vi "Kinematics.vi"() -> ()   [LabVIEW 2024]
panel:
  in  "Lengths":cluster{"L 1":dbl, "L 2":dbl}={"L 1"=80.0, "L 2"=115.0} {"L 2" scale=0.0..200.0; "L 1" scale=0.0..200.0}
  in  "2D Pict origin":cluster{"x":dbl, "y":dbl}={"x"=80.0, "y"=350.0}
  out "2D Picture":picture
  in  "Positions":cluster{dbl, dbl}[](array[cluster]) {"?" format="%.1f"; "?" format="%#.1f"}
  # "mm"
  # "mm"
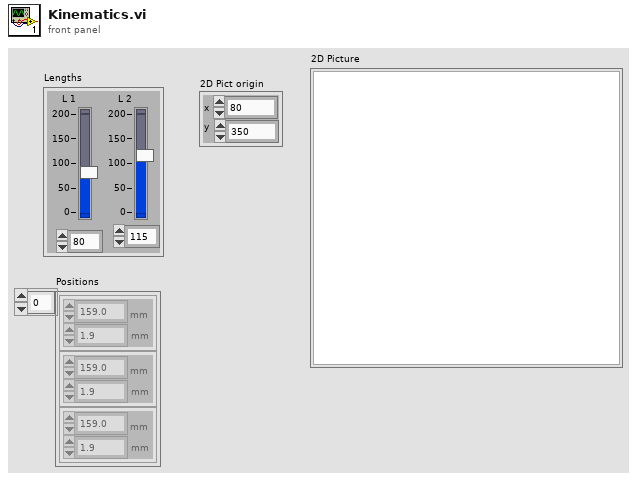
[diagram p1: front panel]
types:
  T1 = cluster{"Width":u16, "Style":enum32{"Solid", "Dash", "Dot", "DashDot", "DashDotDot"}}
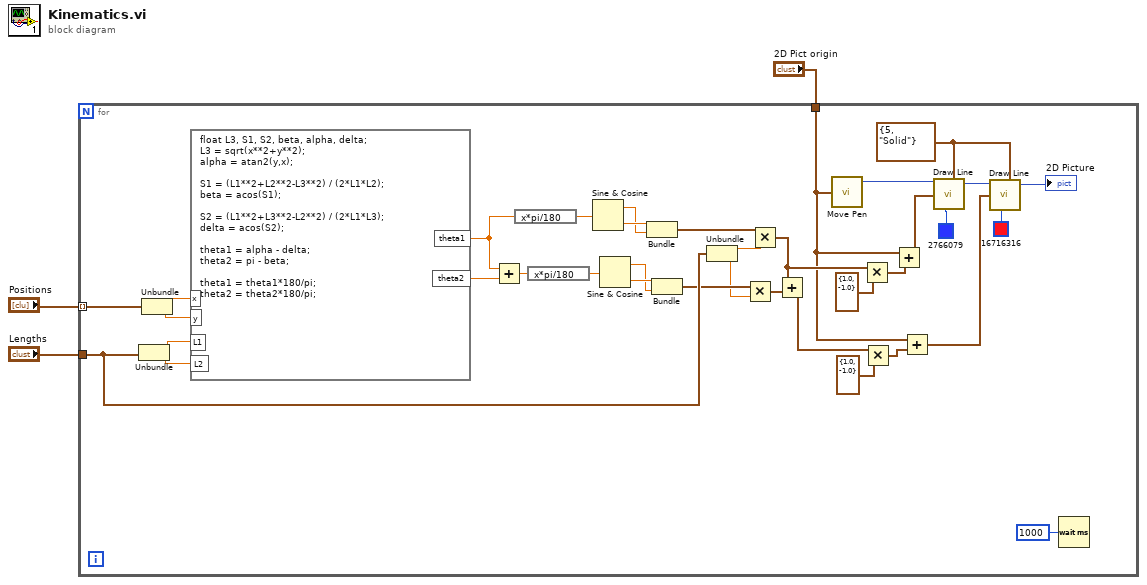
[diagram p0: block diagram]
diagram:
  n1 = for {
    tunnel: "Positions" -> [w37] mode=indexing
    tunnel: "2D Pict origin" -> [w4]
    tunnel: "Lengths" -> [w25]
    w28 = T1 {"Width"=5, "Style"=enum."Solid"} ("pen")
    n2 = Unbundle(w25) -> ("L 1"=w27:dbl, "L 2"=w26:dbl)
    n3 = Unbundle(w37) -> (w39:dbl, w38:dbl)
    n4 = formula code="float L3, S1, S2, beta, alpha, delta;\nL3 = sqrt(x**2+y**2);\nalpha = atan2(y,x);\n\nS1 = (L1**2+L2**2-L3**2) / (2*L1*L2);\nbeta = acos(S1);\n\nS2 = (L1**2+L3**2-L2**2) / (2*L1*L3);\ndelta = acos(S2);\n\ntheta1 = alpha - delta;\ntheta2 = pi - beta;\n\ntheta1 = theta1*180/pi;\ntheta2 = theta2*180/pi;"("L1"=w27, "L2"=w26, "x"=w39, "y"=w38) -> ("theta1"=w24:dbl, "theta2"=w23:dbl)
    n5 = Add(x=w24, y=w23) -> (x+y=w31:dbl)
    n6 = expression code="x*pi/180"(w24) -> (w35:dbl)
    n7 = expression code="x*pi/180"(w31) -> (w34:dbl)
    n8 = Sine & Cosine(0:w35) -> (1:w21:dbl, 2:w22:dbl)
    n9 = Sine & Cosine(0:w34) -> (1:w17:dbl, 2:w18:dbl)
    n10 = Bundle(w22, w21) -> (w20:cluster{dbl, dbl})  [unwired: 1 in]
    n11 = Bundle(w18, w17) -> (w16:cluster{dbl, dbl})  [unwired: 1 in]
    n12 = Unbundle(w25) -> ("L 1"=w19:dbl, "L 2"=w15:dbl)
    n13 = Multiply(x=w16, y=w15) -> (x*y=w11:cluster{dbl, dbl})
    n14 = Multiply(x=w20, y=w19) -> (x*y=w9:cluster{dbl, dbl})
    n15 = Add(x=w9, y=w11) -> (x+y=w7:cluster{dbl, dbl})
    n16 = call <vilib>:"Move Pen.vi"("new position"=w4) -> ("new picture"=w36:picture)  [unwired: 4 in]
    n17 = Multiply(x=w9, y=cluster{dbl, dbl} {1.0, -1.0}) -> (x*y=w10:cluster{dbl, dbl})
    n18 = Multiply(x=w7, y=cluster{dbl, dbl} {1.0, -1.0}) -> (x*y=w6:cluster{dbl, dbl})
    n19 = Add(x=w4, y=w10) -> (x+y=w8:cluster{dbl, dbl})
    n20 = Add(x=w4, y=w6) -> (x+y=w5:cluster{dbl, dbl})
    n21 = call <vilib>:"Draw Line.vi"("picture"=w36, "end point"=w8, "color(black)"=u32 2766079, "pen"=w28) -> ("new picture"=w33:picture)  [unwired: 5 in]
    n22 = call <vilib>:"Draw Line.vi"("picture"=w33, "end point"=w5, "color(black)"=u32 16716316, "pen"=w28) -> ("new picture"=→"2D Picture":picture)  [unwired: 5 in]
    n23 = Wait (ms)(milliseconds to wait=u32 1000) -> ()  [unwired: 1 out]
  }
